vi "PicoScope9300_Example.vi"() -> ()   [LabVIEW 2013]
panel:
  in  "PicoSample3.ICOMRC":refnum<k7>
  out "Plot":cluster{"Xorig":sgl, "Xint":sgl, "Array":sgl[]}(graph)
  in  "Data":bool
  in  "Run":bool
  in  "Stop":bool
  in  "Single":bool
  in  "Command":string
  in  "ON":bool
  out "Response":string
  out "error out":errorcluster
  in  "Send":bool
  in  "OFF":bool
  in  "error in":errorcluster
  # "This VI demostrates the basic steps needed to create Active X client in LabVIEW"
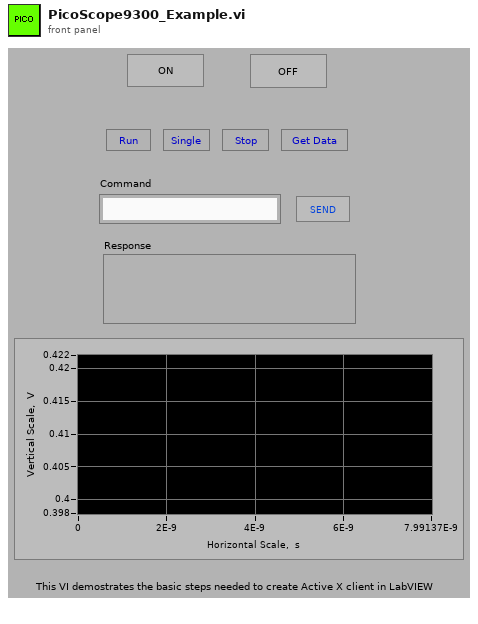
[diagram p1: front panel]
types:
  T1 = cluster{"Xmin":sgl, "Xint":sgl, "Data Array":sgl[]}
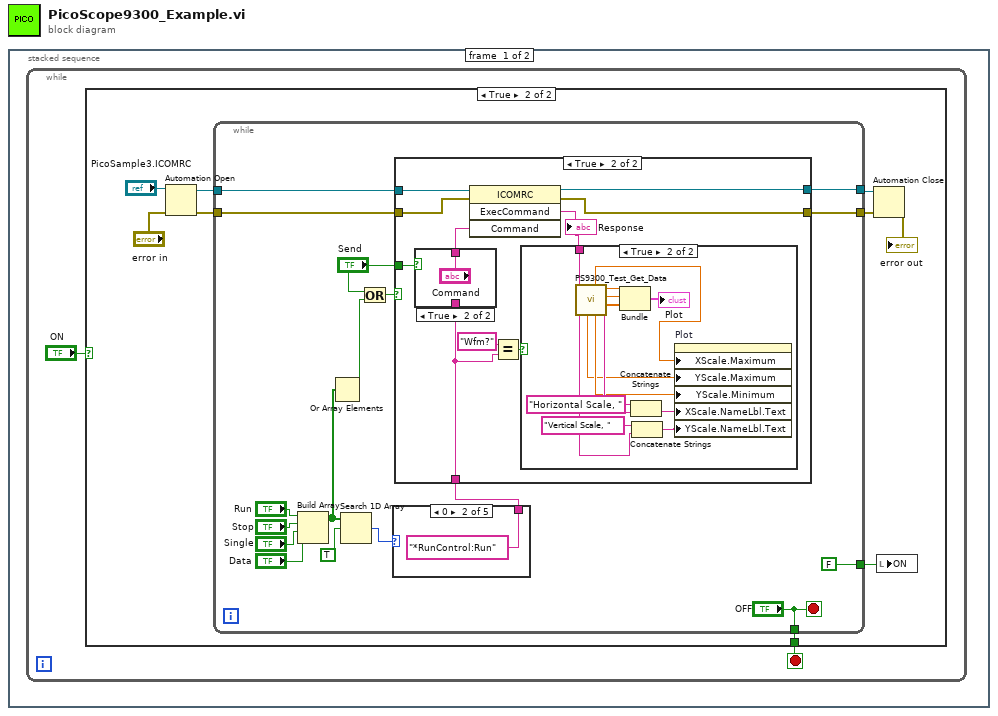
[diagram p0: block diagram]
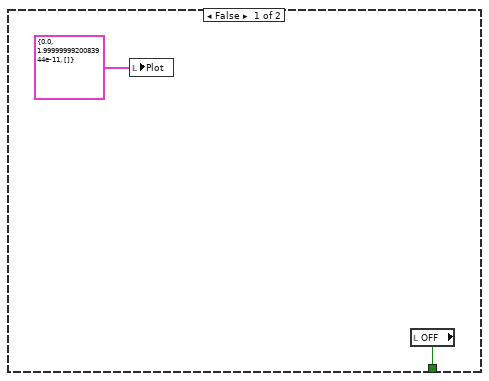
[diagram p2: hidden frame]
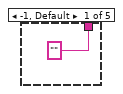
[diagram p3: hidden frame]
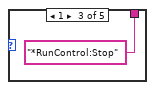
[diagram p4: hidden frame]
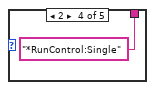
[diagram p5: hidden frame]
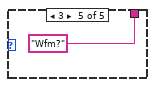
[diagram p6: hidden frame]
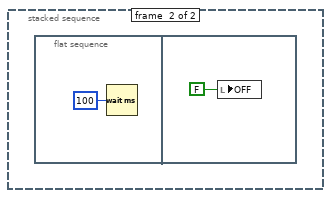
[diagram p10: hidden frame]
diagram:
  n1 = stacked-sequence {
    frame #0 {
      n2 = while {
        stop <- w2 stop-if-true
        n3 = case shown="True" "ON" {
          tunnel: [w3 w7] -> w2
          frame False {
            n4 = local write "Plot"(cluster{"Xorig":sgl, "Xint":sgl, "Array":sgl[]} {"Xorig"=0.0, "Xint"=2e-11, "Array"=[]} ("Single Plot")) -> ()
            n5 = local read "OFF"() -> (w3:bool)
          }
          frame True {
            n6 = Automation Open(error in (no error)="error in", Automation Refnum="PicoSample3.ICOMRC") -> (Automation Refnum=w12:refnum<k7>, error out=w11:errorcluster)  [unwired: 2 in]
            n7 = while {
              tunnel: w12 -> [w30]
              tunnel: w11 -> [w29]
              tunnel: [w28] -> w10
              tunnel: [w27] -> w9
              tunnel: ["OFF"] -> w7
              tunnel: [FALSE] -> w6
              stop <- "OFF" stop-if-true
              n8 = Build Array("Run", "Stop", "Single", "Data") -> (w19:bool[])
              n9 = Or Array Elements(Boolean array=w19) -> (logical OR=w18:bool)
              n10 = Search 1D Array(1D array=w19, element=TRUE) -> (index of element=w15:i32)  [unwired: 1 in]
              n11 = Or(x="Send", y=w18) -> (x .or. y?=w20:bool)
              n12 = case shown="0" w15 {
                tunnel: ["" "*RunControl:Run" "*RunControl:Stop" "*RunControl:Single" "Wfm?"] -> w14
                frame -1, Default {
                }
                frame 0 {
                }
                frame 1 {
                }
                frame 2 {
                }
                frame 3 {
                }
              }
              n13 = case shown="True" w20 {
                tunnel: w30 -> [w37 w47]
                tunnel: w29 -> [w36 w46]
                tunnel: [w37 w45] -> w28
                tunnel: [w36 w44] -> w27
                tunnel: w14 -> [_ w40]
                tunnel: "Send" -> [_ w42]
                frame False {
                }
                frame True {
                  n14 = case shown="True" w42 {
                    tunnel: [w62 "Command"] -> w43
                    tunnel: w40 -> [w62 _]
                    frame False {
                    }
                    frame True {
                    }
                  }
                  n15 = invoke class="ICOMRC" method="ExecCommand"(reference=w47, error in=w46, "Command"=w43) -> (reference out=w45:refnum<k7>, error out=w44:errorcluster, "ExecCommand"=w38:string)  [unwired: 1 in, 1 out]
                  "Response" <- w38
                  n16 = Equal?(x="Wfm?", y=w40) -> (x = y?=w41:bool)
                  n17 = case shown="True" w41 {
                    tunnel: w38 -> [_ w61]
                    frame False {
                    }
                    frame True {
                      n18 = call "PS9300_Test_Get_Data.vi"("ExecCommand"=w61) -> ("XU"=w56:string, "Data Array"=w58:sgl[], "Xint"=w51:sgl, "Xmin"=w59:sgl, "Ymin"=w50:sgl, "Xmax"=w48:sgl, "Ymax"=w49:sgl, "YU"=w53:string)  [unwired: 2 in, 1 out]
                      n19 = Bundle("Xmin"=w59, "Xint"=w51, "Data Array"=w58) -> (→"Plot":T1)  [unwired: 1 in]
                      n20 = Concatenate Strings("Horizontal Scale, " ("string"), w56) -> (w55:string)
                      n21 = Concatenate Strings("Vertical Scale, " ("string"), w53) -> (w52:string)
                      n22 = property on="Plot" class="WFGraph (strict)"("XScale.Maximum"=w48, "YScale.Maximum"=w49, "YScale.Minimum"=w50, "XScale.NameLbl.Text"=w55, "YScale.NameLbl.Text"=w52) -> ()  [unwired: 2 in, 2 out]
                    }
                  }
                }
              }
            }
            n23 = Automation Close(3:w9, 5:w10) -> (0:→"error out":errorcluster)
            n24 = local write "ON"(w6) -> ()
          }
        }
      }
    }
    frame #1 {
      n25 = flat-sequence {
        frame #0 {
          n26 = Wait (ms)(milliseconds to wait=u32 100) -> ()  [unwired: 1 out]
        }
        frame #1 {
          n27 = local write "OFF"(FALSE ("stop")) -> ()
        }
      }
    }
  }
